vi "test Acyclic Tx Encode Parameters into Words for Labels in a Channel.vi"(8 "error in":errorcluster, 11 "TestCase in":refnum<class "Engine.lvclass">) -> (0 "error out":errorcluster, 3 "TestCase out":refnum<class "Engine.lvclass">)   [LabVIEW 2020, in "Engine.lvclass"]
uses:
  Engine.lvclass
  Shared/RT Label Settings.ctl
  Shared/Label.ctl
  Shared/RT Parameters.ctl
  Shared/Parameter Definition.ctl
  <vilib>/NI/NI VeriStand Encoding and Decoding/Encoding.ctl
  <vilib>/NI VeriStand/Custom Device API/Custom Device Item Ref.ctl
  Shared/Transfer Type.ctl
  <vilib>/NI VeriStand/Custom Device API/Data Reference.ctl
  Hardware API/Data Word with Trigger.ctl
  <vilib>/addons/_JKI Toolkits/VI Tester/TestCase.llb/TestCase.lvclass
  <vilib>/NI VeriStand/Custom Device API/Custom Device API.lvlib
  <vilib>/NI/NI VeriStand Encoding and Decoding/Encoding and Decoding.lvlib
  Engine/Implementation/Tx Acyclic Labels Execution Unit/Tx Acyclic Labels Execution Unit.lvclass
  Hardware API/AIM ARINC 429 Hardware API.lvlib
  C:/Program Files (x86)/National Instruments/LabVIEW 2020/vi.lib/addons/_JKI Toolkits/VI Tester/TestCase.llb/TestCase.lvclass
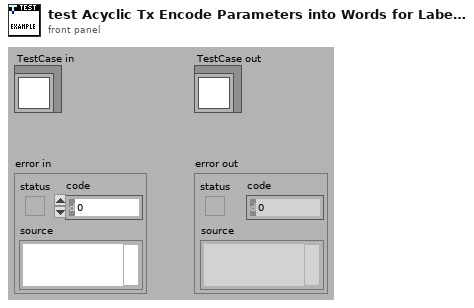
[diagram p1: front panel]
types:
  T1 = typedef "RT Label Settings.ctl" = cluster{"Name":string, "xmlName":string, "label":T2, "transfer period":u32, "SDI_Enabled":bool, "SDI":u8, "parameter driver data":T3, "transfer type":T7, "has timestamp?":bool, "Label Disable/Trigger Channel Reference":T6, "Message Handle":u64, "Initialized?":bool, "Word Initial Raw Value":u32, "Label Timestamp Channel Data Reference":T8, "disabled":bool}
  T2 = typedef "Label.ctl" = u8
  T3 = typedef "RT Parameters.ctl" = cluster{"parameter definitions":T4[], "Tx parameter refs":T6[]}
  T4 = typedef "Parameter Definition.ctl" = cluster{"start index":i32, "size":i32, "encoding":T5, "signed":bool, "scale multiplier":dbl, "scale offset":dbl, "default value":dbl}
  T5 = typedef "Encoding and Decoding.lvlib/Encoding.ctl" = enum16{"BNR", "BCD", "Discrete"}
  T6 = typedef "Custom Device API.lvlib/Custom Device Item Ref.ctl" = u64
  T7 = typedef "Transfer Type.ctl" = enum16{"Scheduled", "Acyclic", "Block", "Strobe"}
  T8 = typedef "Custom Device API.lvlib/Data Reference.ctl" = i32
  T9 = typedef "AIM ARINC 429 Hardware API.lvlib/Data Word with Trigger.ctl" = cluster{"Trigger":bool, "Data Word":u32}
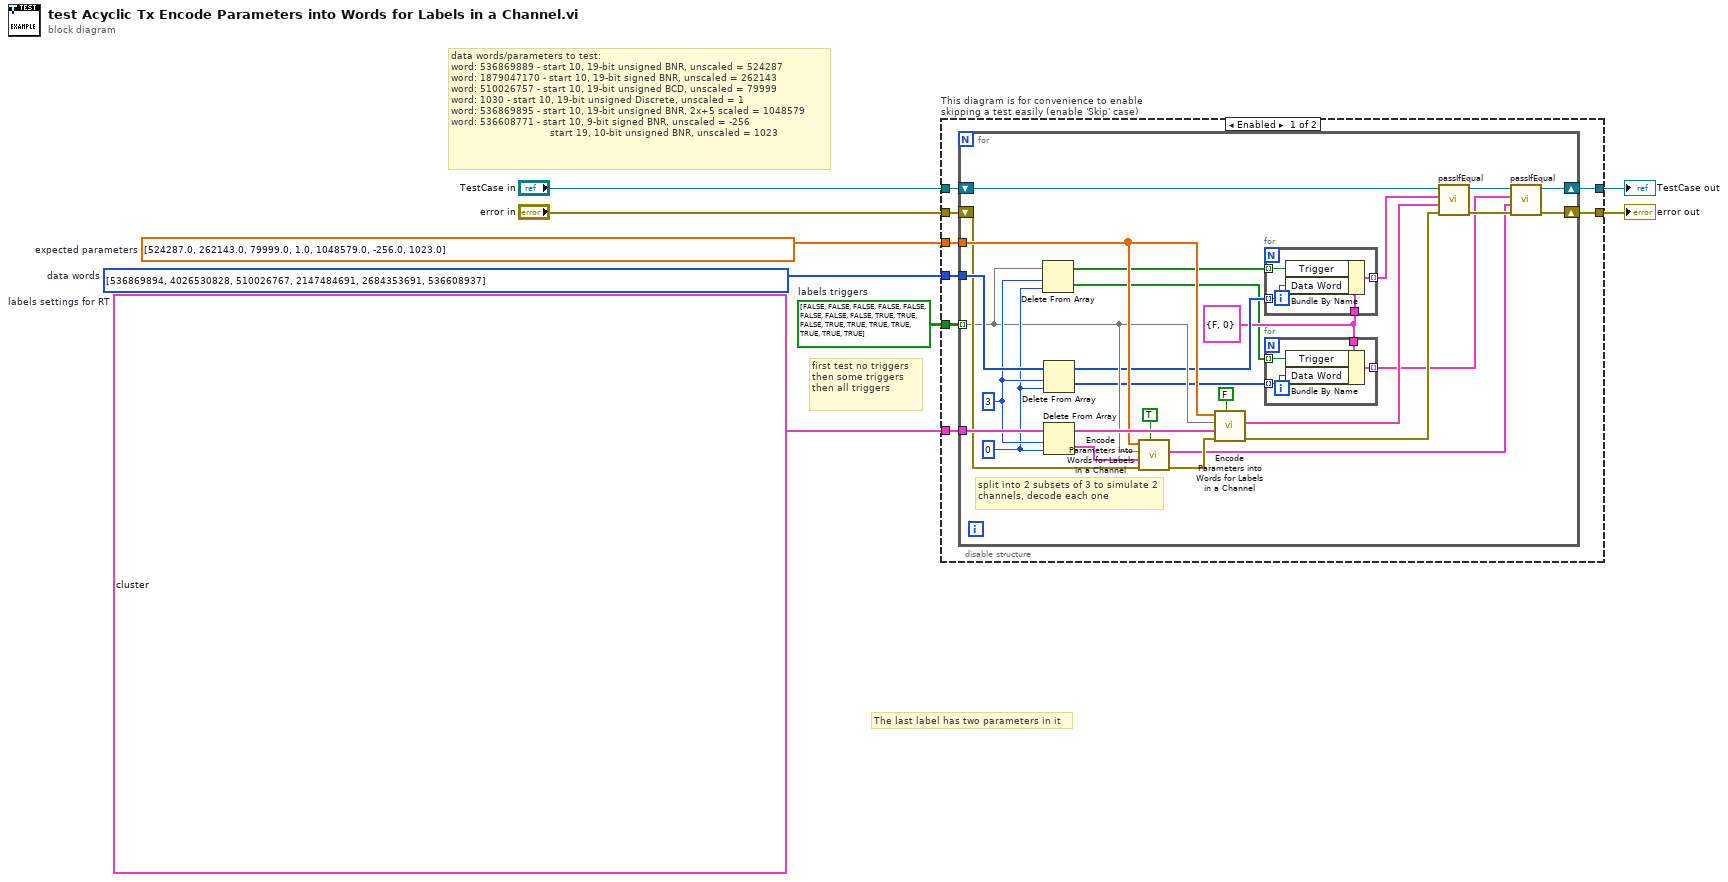
[diagram p0: block diagram]
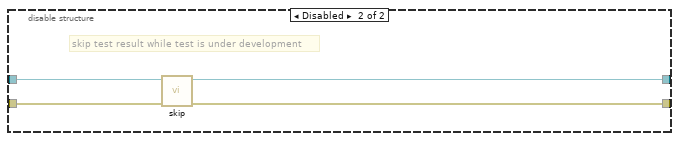
[diagram p2: hidden frame]
diagram:
  w1 = bool[][] [[FALSE, FALSE, FALSE, FALSE, FALSE, FALSE], [FALSE, FALSE, TRUE, TRUE, FALSE, TRUE], [TRUE, TRUE, TRUE, TRUE, TRUE, TRUE]]  # labels triggers
  w3 = dbl[] [524287.0, 262143.0, 79999.0, 1.0, 1048579.0, -256.0, 1023.0]  # expected parameters
  w4 = T1[] [{"Name"="", "xmlName"="", "label"=6, "transfer period"=10, "SDI_Enabled"=FALSE, "SDI"=0, "parameter driver data"={"parameter definitions"=[{"start index"=10, "size"=19, "encoding"=enum."BNR", "signed"=FALSE, "scale multiplier"=1.0, "scale offset"=0.0, "default value"=0.0}], "Tx parameter refs"=[]}, "transfer type"=enum."Acyclic", "has timestamp?"=FALSE, "Label Disable/Trigger Channel Reference"=0, "Message Handle"=0, "Initialized?"=FALSE, "Word Initial Raw Value"=0, "Label Timestamp Channel Data Reference"=0, "disabled"=FALSE}, {"Name"="", "xmlName"="", "label"=12, "transfer period"=10, "SDI_Enabled"=FALSE, "SDI"=0, "parameter driver data"={"parameter definitions"=[{"start index"=10, "size"=19, "encoding"=enum."BNR", "signed"=TRUE, "scale multiplier"=1.0, "scale offset"=0.0, "default value"=0.0}], "Tx parameter refs"=[]}, "transfer type"=enum."Acyclic", "has timestamp?"=FALSE, "Label Disable/Trigger Channel Reference"=0, "Message Handle"=0, "Initialized?"=FALSE, "Word Initial Raw Value"=0, "Label Timestamp Channel Data Reference"=0, "disabled"=FALSE}, {"Name"="", "xmlName"="", "label"=15, "transfer period"=10, "SDI_Enabled"=FALSE, "SDI"=0, "parameter driver data"={"parameter definitions"=[{"start index"=10, "size"=19, "encoding"=enum."BCD", "signed"=FALSE, "scale multiplier"=1.0, "scale offset"=0.0, "default value"=0.0}], "Tx parameter refs"=[]}, "transfer type"=enum."Acyclic", "has timestamp?"=FALSE, "Label Disable/Trigger Channel Reference"=0, "Message Handle"=0, "Initialized?"=FALSE, "Word Initial Raw Value"=0, "Label Timestamp Channel Data Reference"=0, "disabled"=FALSE}, {"Name"="", "xmlName"="", "label"=19, "transfer period"=10, "SDI_Enabled"=FALSE, "SDI"=0, "parameter driver data"={"parameter definitions"=[{"start index"=10, "size"=19, "encoding"=enum."Discrete", "signed"=FALSE, "scale multiplier"=1.0, "scale offset"=0.0, "default value"=0.0}], "Tx parameter refs"=[]}, "transfer type"=enum."Acyclic", "has timestamp?"=FALSE, "Label Disable/Trigger Channel Reference"=0, "Message Handle"=0, "Initialized?"=FALSE, "Word Initial Raw Value"=0, "Label Timestamp Channel Data Reference"=0, "disabled"=FALSE}, {"Name"="", "xmlName"="", "label"=155, "transfer period"=10, "SDI_Enabled"=FALSE, "SDI"=0, "parameter driver data"={"parameter definitions"=[{"start index"=10, "size"=19, "encoding"=enum."BNR", "signed"=FALSE, "scale multiplier"=2.0, "scale offset"=5.0, "default value"=0.0}], "Tx parameter refs"=[]}, "transfer type"=enum."Acyclic", "has timestamp?"=FALSE, "Label Disable/Trigger Channel Reference"=0, "Message Handle"=0, "Initialized?"=FALSE, "Word Initial Raw Value"=0, "Label Timestamp Channel Data Reference"=0, "disabled"=FALSE}, {"Name"="", "xmlName"="", "label"=169, "transfer period"=10, "SDI_Enabled"=FALSE, "SDI"=0, "parameter driver data"={"parameter definitions"=[{"start index"=10, "size"=9, "encoding"=enum."BNR", "signed"=TRUE, "scale multiplier"=1.0, "scale offset"=0.0, "default value"=0.0}, {"start index"=19, "size"=10, "encoding"=enum."BNR", "signed"=FALSE, "scale multiplier"=1.0, "scale offset"=0.0, "default value"=0.0}], "Tx parameter refs"=[]}, "transfer type"=enum."Acyclic", "has timestamp?"=FALSE, "Label Disable/Trigger Channel Reference"=0, "Message Handle"=0, "Initialized?"=FALSE, "Word Initial Raw Value"=0, "Label Timestamp Channel Data Reference"=0, "disabled"=FALSE}]  # labels settings for RT
  w5 = u32[] [536869894, 4026530828, 510026767, 2147484691, 2684353691, 536608937]  # data words
  # "first test no triggers\nthen some triggers\nthen all triggers"
  # "The last label has two parameters in it"
  # "for visibility, irrelevant label settings are minimized in this constant"
  # "data words/parameters to test:\nword: 536869889 - start 10, 19-bit unsigned BNR, unscaled = 524287\nword: 1879047170 - start 10, 19-bit signed BNR, unscaled = 262143\nword: 510026757 - start 10, 19-bit unsigned BCD, unscaled = 79999\nword: 1030 - start 10, 19-bit unsigned Discrete, unscaled = 1\nword: 536869895 - start 10, 19-bit unsigned BNR, 2x+5 scaled = 1048579 \nword: 536608771 - start 10, 9-bit signed BNR, unscaled = -256\n                                 start 19, 10-bit unsigned BNR, unscaled = 1023"
  n1 = disable-structure "This diagram is for convenience to enable skipping a test easily (enable 'Skip' case)" shown="Enabled" {
    disable-tunnel: "TestCase in" -> [w14 w55]
    disable-tunnel: [w13 w53] -> w2
    disable-tunnel: [w12 w54] -> w7
    disable-tunnel: "error in" -> [w9 w52]
    disable-tunnel: w5 -> [w15 _]
    disable-tunnel: w4 -> [w16 _]
    disable-tunnel: w3 -> [w11 _]
    disable-tunnel: w1 -> [w10 _]
    frame Enabled {
      n2 = for {
        tunnel: w16 -> [w43]
        tunnel: w15 -> [w42]
        tunnel: w11 -> [w37]
        shift-right: [w26] -> w13
        shift-left: w14 -> [w41]
        tunnel: w10 -> [w30] mode=indexing
        shift-right: [w27] -> w12
        shift-left: w9 -> [w33]
        w21 = T9 {"Trigger"=FALSE, "Data Word"=0} ("data with triggers out")
        w31 = 0 ("index")
        w32 = 3 ("length")
        # "split into 2 subsets of 3 to simulate 2 channels, decode each one"
        n3 = Delete From Array(array=w30, length=w32, index=w31) -> (deleted portion=w20:bool[], array with subset deleted=w25:bool[])
        n4 = Delete From Array(array=w42, length=w32, index=w31) -> (deleted portion=w19:u32[], array with subset deleted=w24:u32[])
        n5 = Delete From Array(array=w43, length=w32, index=w31) -> (deleted portion=w40:T1[], array with subset deleted=w38:T1[])
        n6 = call "Encode Parameters into Words for Labels in a Channel.vi"("reset index"=TRUE, "error in (no error)"=w33, "labels settings for RT in"=w40, "Triggers in"=w30, "Parameter Values in"=w37) -> ("error out"=w34:errorcluster, "data with triggers out"=w17:T9[])  [unwired: 5 in]
        n7 = call "Encode Parameters into Words for Labels in a Channel.vi"("reset index"=FALSE, "error in (no error)"=w34, "labels settings for RT in"=w38, "Triggers in"=w30, "Parameter Values in"=w37) -> ("error out"=w35:errorcluster, "data with triggers out"=w22:T9[])  [unwired: 5 in]
        n8 = for {
          tunnel: w25 -> [w50] mode=indexing
          tunnel: w24 -> [w49] mode=indexing
          tunnel: w21 -> [w51]
          tunnel: [w48] -> w23 mode=indexing
          n9 = Bundle By Name(cluster=w51, "Trigger"=w50, "Data Word"=w49) -> (w48:T9)
        }
        n10 = for {
          tunnel: w20 -> [w46] mode=indexing
          tunnel: w19 -> [w45] mode=indexing
          tunnel: w21 -> [w47]
          tunnel: [w44] -> w18 mode=indexing
          n11 = Bundle By Name(cluster=w47, "Trigger"=w46, "Data Word"=w45) -> (w44:T9)
        }
        n12 = call-dynamic "passIfEqual.vi"("error in (no error)"=w35, "y"=w22, "x"=w23, "TestCase in"=w41) -> ("error out"=w29:errorcluster, "TestCase out"=w28:refnum<class "Engine.lvclass">)  [unwired: 6 in]
        n13 = call-dynamic "passIfEqual.vi"("error in (no error)"=w29, "y"=w17, "x"=w18, "TestCase in"=w28) -> ("error out"=w27:errorcluster, "TestCase out"=w26:refnum<class "Engine.lvclass">)  [unwired: 6 in]
      }
    }
    frame Disabled {
      # "skip test result while test is under development"
      n14 = call <vilib>:"skip.vi"("error in (no error)"=w52, "TestCase in"=w55) -> ("error out"=w54:errorcluster, "TestCase out"=w53:refnum<class "Engine.lvclass">)  [unwired: 8 in]
    }
  }
  "error out" <- w7
  "TestCase out" <- w2
